vi "Configure Trigger (Logic).vi"(0 "VISA resource name":refnum<visa-resource-name>, 1 "Pattern Input":T1={"Channel 1 Logic Input (2: X)"=2, "Channel 2 Logic Input (2: X)"=2, "Channel 3 Logic Input (2: X)"=2, "Channel 4 Logic Input (2: X)"=2, "RF Channel Logic Input (2: X)"=2} {"RF Channel Logic Input (2: X)" items=["High", "Low", "X"]; "Channel 4 Logic Input (2: X)" items=["High", "Low", "X"]; "Channel 3 Logic Input (2: X)" items=["High", "Low", "X"]; "Channel 2 Logic Input (2: X)" items=["High", "Low", "X"]; "Channel 1 Logic Input (2: X)" items=["High", "Low", "X"]}, 2 "RF Logic Threshold (-22dBm)":dbl=-22.0 min=-40.0 max=10.0 step=1.0 format="%#_g dBm", 5 "Function (0: AND)":u16(ring) items=["AND", "OR", "NAND", "NOR"], 7 "Clock Source (1: Channel 1)":u16(ring)=1 items=["None", "Channel 1", "Channel 2", "Channel 3", "Channel 4", "Digital Channel 0", "Digital Channel 1", "Digital Channel 2", "Digital Channel 3", "Digital Channel 4", "Digital Channel 5", "Digital Channel 6", "Digital Channel 7", "Digital Channel 8", "Digital Channel 9", "Digital Channel 10", "Digital Channel 11", "Digital Channel 12", "Digital Channel 13", "Digital Channel 14", "Digital Channel 15", "RF"], 9 "Clock Polarity (0: Rising)":u16(ring) items=["Rising", "Falling"], 11 "error in (no error)":errorcluster, 12 "Trigger Condition (0: True)":u16(ring) items=["True", "False", "Less Than", "More Than", "Equal", "Not Equal"], 13 "Delta Time (4.0ns)":dbl=4e-09) -> (4 "VISA resource name out":refnum<visa-resource-name>, 15 "error out":errorcluster)   [LabVIEW 2013, in "Tektronix DPO MSO 2000 4000 Series.lvlib"]
doc: "Configures logic trigger settings for an oscilloscope."
uses:
  Tektronix DPO MSO 2000 4000 Series.lvlib
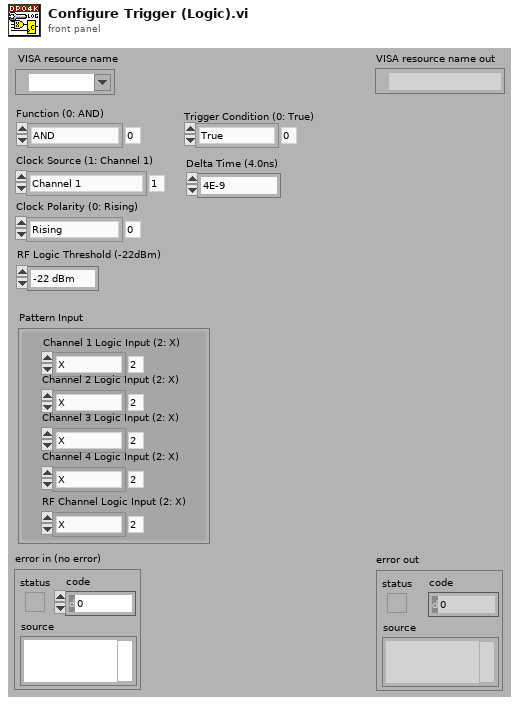
[diagram p1: front panel]
types:
  T1 = cluster{"Channel 1 Logic Input (2: X)":u16, "Channel 2 Logic Input (2: X)":u16, "Channel 3 Logic Input (2: X)":u16, "Channel 4 Logic Input (2: X)":u16, "RF Channel Logic Input (2: X)":u16}
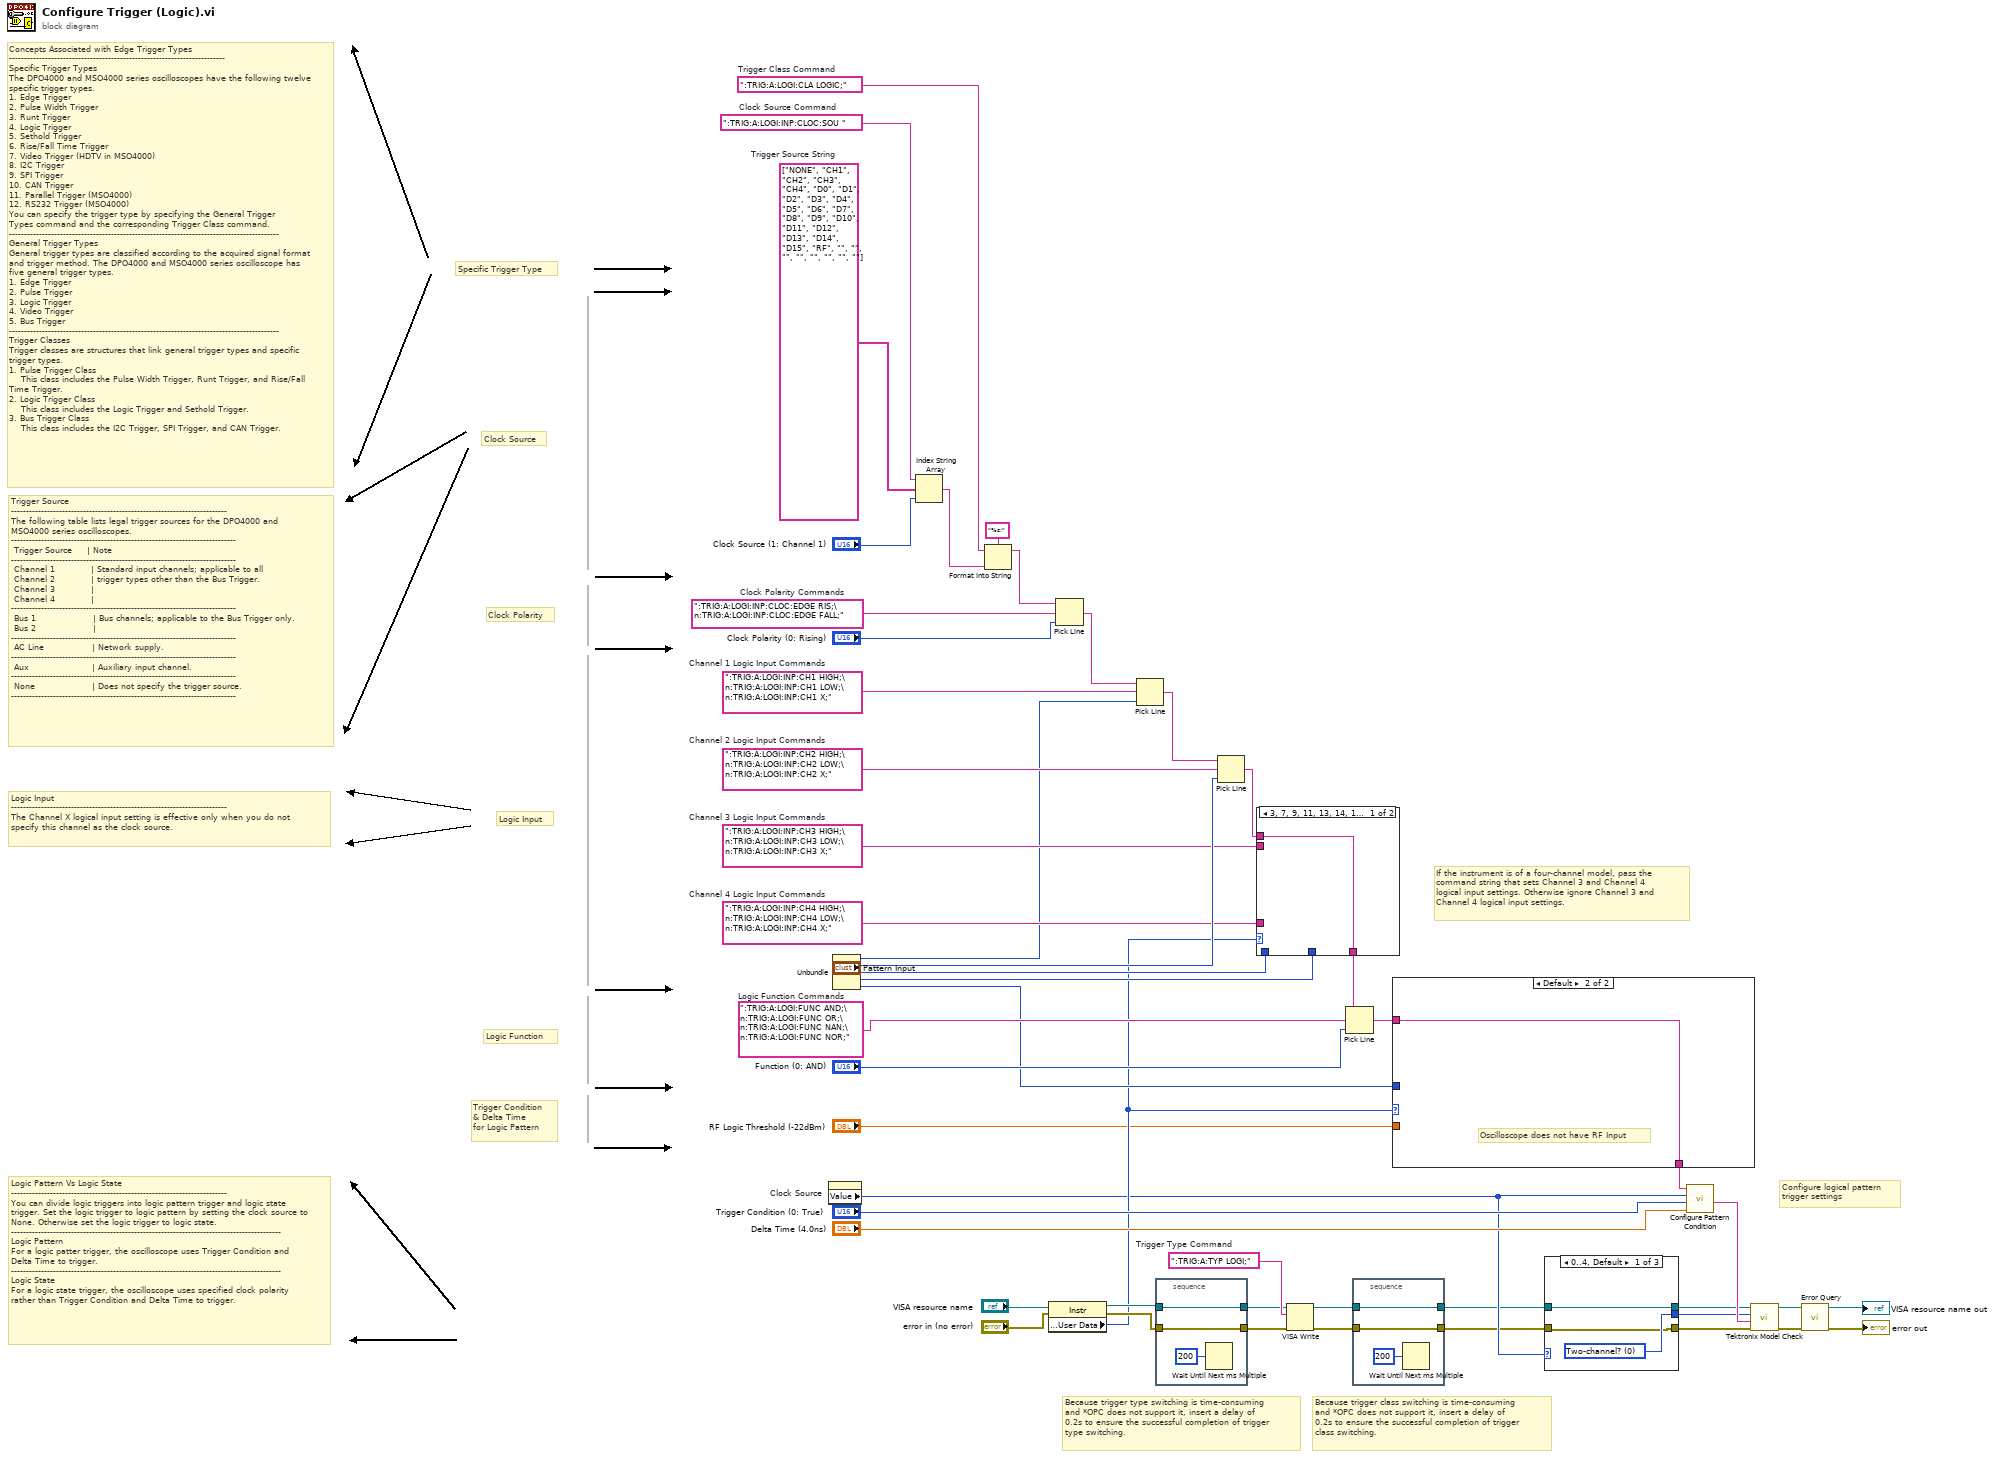
[diagram p0: block diagram]
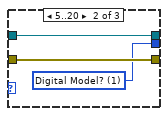
[diagram p2: hidden frame]
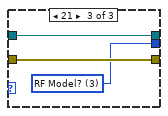
[diagram p3: hidden frame]
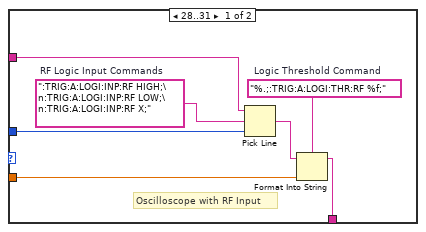
[diagram p4: hidden frame]
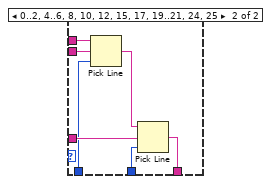
[diagram p5: hidden frame]
diagram:
  w25 = string[] ["NONE", "CH1", "CH2", "CH3", "CH4", "D0", "D1", "D2", "D3", "D4", "D5", "D6", "D7", "D8", "D9", "D10", "D11", "D12", "D13", "D14", "D15", "RF", "", "", "", "", "", "", "", ""]  # Trigger Source String
  w35 = ":TRIG:A:LOGI:INP:CH4 HIGH;\n:TRIG:A:LOGI:INP:CH4 LOW;\n:TRIG:A:LOGI:INP:CH4 X;"  # Channel 4 Logic Input Commands
  w36 = ":TRIG:A:LOGI:INP:CH3 HIGH;\n:TRIG:A:LOGI:INP:CH3 LOW;\n:TRIG:A:LOGI:INP:CH3 X;"  # Channel 3 Logic Input Commands
  w40 = ":TRIG:A:LOGI:INP:CH2 HIGH;\n:TRIG:A:LOGI:INP:CH2 LOW;\n:TRIG:A:LOGI:INP:CH2 X;"  # Channel 2 Logic Input Commands
  w41 = ":TRIG:A:LOGI:INP:CH1 HIGH;\n:TRIG:A:LOGI:INP:CH1 LOW;\n:TRIG:A:LOGI:INP:CH1 X;"  # Channel 1 Logic Input Commands
  w44 = ":TRIG:A:LOGI:FUNC AND;\n:TRIG:A:LOGI:FUNC OR;\n:TRIG:A:LOGI:FUNC NAN;\n:TRIG:A:LOGI:FUNC NOR;"  # Logic Function Commands
  w46 = ":TRIG:A:LOGI:INP:CLOC:EDGE RIS;\n:TRIG:A:LOGI:INP:CLOC:EDGE FALL;"  # Clock Polarity Commands
  w48 = ":TRIG:A:LOGI:INP:CLOC:SOU "  # Clock Source Command
  w24 = ":TRIG:A:LOGI:CLA LOGIC;"  # Trigger Class Command
  w51 = ":TRIG:A:TYP LOGI;"  # Trigger Type Command
  # "Trigger Source\n------------------------------------------------------------------------\nThe following table lists legal trigger sources for the DPO4000 and MSO4000 series oscilloscopes.\n---------------------------------------------------------------------------\n Trigger Source     | Note                                                           \n---------------------------------------------------------------------------\n Channel 1            | Standard input channels; applicable to all      \n Channel 2            | trigger types other than the Bus Trigger.         \n Channel 3            |     \n Channel 4            |\n---------------------------------------------------------------------------\n Bus 1                   | Bus channels; applicable to the Bus Trigger only.\n Bus 2                   | \n---------------------------------------------------------------------------\n AC Line                | Network supply.\n---------------------------------------------------------------------------\n Aux                     | Auxiliary input channel.\n---------------------------------------------------------------------------\n None                   | Does not specify the trigger source.\n---------------------------------------------------------------------------"
  # "Concepts Associated with Edge Trigger Types\n------------------------------------------------------------------------\nSpecific Trigger Types\nThe DPO4000 and MSO4000 series oscilloscopes have the following twelve specific trigger types.\n1. Edge Trigger\n2. Pulse Width Trigger\n3. Runt Trigger\n4. Logic Trigger\n5. Sethold Trigger\n6. Rise/Fall Time Trigger\n7. Video Trigger (HDTV in MSO4000)\n8. I2C Trigger\n9. SPI Trigger\n10. CAN Trigger\n11. Parallel Trigger (MSO4000)\n12. RS232 Trigger (MSO4000)\nYou can specify the trigger type by specifying the General Trigger \nTypes command and the corresponding Trigger Class command.\n------------------------------------------------------------------------------------------\nGeneral Trigger Types \nGeneral trigger types are classified according to the acquired signal format and trigger method. The DPO4000 and MSO4000 series oscilloscope has five general trigger types.\n1. Edge Trigger\n2. Pulse Trigger\n3. Logic Trigger\n4. Video Trigger\n5. Bus Trigger\n------------------------------------------------------------------------------------------\nTrigger Classes\nTrigger classes are structures that link general trigger types and specific trigger types.\n1. Pulse Trigger Class\n    This class includes the Pulse Width Trigger, Runt Trigger, and Rise/Fall Time Trigger.\n2. Logic Trigger Class\n    This class includes the Logic Trigger and Sethold Trigger.\n3. Bus Trigger Class\n    This class includes the I2C Trigger, SPI Trigger, and CAN Trigger."
  # "Because trigger type switching is time-consuming\nand *OPC does not support it, insert a delay of\n0.2s to ensure the successful completion of trigger\ntype switching."
  # "Because trigger class switching is time-consuming\nand *OPC does not support it, insert a delay of\n0.2s to ensure the successful completion of trigger\nclass switching."
  # "Configure logical pattern\ntrigger settings"
  # "If the instrument is of a four-channel model, pass the\ncommand string that sets Channel 3 and Channel 4\nlogical input settings. Otherwise ignore Channel 3 and\nChannel 4 logical input settings."
  # "Logic Pattern Vs Logic State\n------------------------------------------------------------------------\nYou can divide logic triggers into logic pattern trigger and logic state trigger. Set the logic trigger to logic pattern by setting the clock source to None. Otherwise set the logic trigger to logic state.\n------------------------------------------------------------------------------------------\nLogic Pattern\nFor a logic patter trigger, the oscilloscope uses Trigger Condition and Delta Time to trigger.\n------------------------------------------------------------------------------------------\nLogic State\nFor a logic state trigger, the oscilloscope uses specified clock polarity rather than Trigger Condition and Delta Time to trigger."
  # "Logic Input\n------------------------------------------------------------------------\nThe Channel X logical input setting is effective only when you do not specify this channel as the clock source."
  # "Trigger Condition\n& Delta Time \nfor Logic Pattern"
  # "Logic Function"
  # "Logic Input"
  # "Clock Polarity"
  # "Clock Source"
  # "Specific Trigger Type"
  n1 = property on="Clock Source" class="Ring (strict)"() -> ("Value"=w6:u16)  [unwired: 2 in, 2 out]
  n2 = Unbundle("Pattern Input") -> ("Channel 1 Logic Input (2: X)"=w16:u16, "Channel 2 Logic Input (2: X)"=w38:u16, "Channel 3 Logic Input (2: X)"=w34:u16, "Channel 4 Logic Input (2: X)"=w33:u16, "RF Channel Logic Input (2: X)"=w10:u16)
  n3 = Index String Array(1:"Clock Source (1: Channel 1)", 2:w25, 3:w48) -> (0:w23:string)
  n4 = Format Into String(format string="%s;", initial string=w24, w23) -> (resulting string=w45:string)  [unwired: 1 in, 1 out]
  n5 = property class="Instr"(reference="VISA resource name", error in="error in (no error)") -> (reference out=w21:refnum<visa-resource-name>, error out=w20:errorcluster, "General Settings:User Data"=w9:u32)
  n6 = Pick Line(string ("")=w45, multi-line string=w46, line index="Clock Polarity (0: Rising)") -> (output string=w22:string)
  n7 = Pick Line(string ("")=w22, multi-line string=w41, line index=w16) -> (output string=w39:string)
  n8 = stacked-sequence {
    tunnel: w21 -> [w53]
    tunnel: [w53] -> w50
    tunnel: w20 -> [w52]
    tunnel: [w52] -> w49
    frame #0 {
      n9 = Wait Until Next ms Multiple(millisecond multiple=u32 200) -> ()  [unwired: 1 out]
    }
  }
  n10 = Pick Line(string ("")=w39, multi-line string=w40, line index=w38) -> (output string=w37:string)
  n11 = case shown="3, 7, 9, 11, 13, 14, 16, 18, 22, 23, 26, 27, Default" w9 {
    tunnel: w37 -> [w55 w62]
    tunnel: w36 -> [_ w61]
    tunnel: w35 -> [_ w59]
    tunnel: w34 -> [_ w58]
    tunnel: w33 -> [_ w57]
    tunnel: [w55 w56] -> w17
    frame 3, 7, 9, 11, 13, 14, 16, 18, 22, 23, 26, 27, Default {
    }
    frame 0..2, 4..6, 8, 10, 12, 15, 17, 19..21, 24, 25 {
      n12 = Pick Line(string ("")=w62, multi-line string=w61, line index=w58) -> (output string=w60:string)
      n13 = Pick Line(string ("")=w60, multi-line string=w59, line index=w57) -> (output string=w56:string)
    }
  }
  n14 = VISA Write(VISA resource name=w50, write buffer=w51, error in (no error)=w49) -> (VISA resource name out=w32:refnum<visa-resource-name>, error out=w31:errorcluster)  [unwired: 1 out]
  n15 = Pick Line(string ("")=w17, multi-line string=w44, line index="Function (0: AND)") -> (output string=w11:string)
  n16 = stacked-sequence {
    tunnel: w32 -> [w64]
    tunnel: [w64] -> w5
    tunnel: w31 -> [w63]
    tunnel: [w63] -> w3
    frame #0 {
      n17 = Wait Until Next ms Multiple(millisecond multiple=u32 200) -> ()  [unwired: 1 out]
    }
  }
  n18 = case shown="Default" w9 {
    tunnel: w11 -> [w70 w73]
    tunnel: w10 -> [w71 _]
    tunnel: "RF Logic Threshold (-22dBm)" -> [w69 _]
    tunnel: [w66 w73] -> w7
    frame 28..31 {
      w67 = "%.;:TRIG:A:LOGI:THR:RF %f;"  # Logic Threshold Command
      w72 = ":TRIG:A:LOGI:INP:RF HIGH;\n:TRIG:A:LOGI:INP:RF LOW;\n:TRIG:A:LOGI:INP:RF X;"  # RF Logic Input Commands
      # "Oscilloscope with RF Input"
      n19 = Pick Line(string ("")=w70, multi-line string=w72, line index=w71) -> (output string=w68:string)
      n20 = Format Into String(format string=w67, initial string=w68, w69) -> (resulting string=w66:string)  [unwired: 1 in, 1 out]
    }
    frame Default {
      # "Oscilloscope does not have RF Input"
    }
  }
  n21 = case shown="0..4, Default" w6 {
    tunnel: w5 -> [w74 w79 w82]
    tunnel: [w74 w79 w82] -> w4
    tunnel: w3 -> [w75 w78 w81]
    tunnel: [w75 w78 w81] -> w2
    tunnel: [w76 w77 w80] -> w1
    frame 0..4, Default {
      w76 = u16 0 items=["Two-channel?", "Digital Model?", "Four-channel?", "RF Model?"] ("Oscilloscope Model Tests (3: RF Model?)")
    }
    frame 5..20 {
      w77 = u16 1 items=["Two-channel?", "Digital Model?", "Four-channel?", "RF Model?"] ("Oscilloscope Model Tests (3: RF Model?)")
    }
    frame 21 {
      w80 = u16 3 items=["Two-channel?", "Digital Model?", "Four-channel?", "RF Model?"] ("Oscilloscope Model Tests (3: RF Model?)")
    }
  }
  n22 = call "Configure Pattern Condition.vi"("Delta Time (2.5E-9)"="Delta Time (4.0ns)", "Trigger Condition (0: True)"="Trigger Condition (0: True)", "Clock Source (0: Channel 1)"=w6, "Input Command String"=w7) -> ("Output Command String"=w14:string)  [unwired: 7 in]
  n23 = call "Tektronix Model Check.vi"("error in (no error)"=w2, "Command String"=w14, "Oscilloscope Model Tests (3: RF Model?)"=w1, "VISA resource name"=w4) -> ("error out"=w12:errorcluster, "VISA resource name out"=w13:refnum<visa-resource-name>)  [unwired: 6 in]
  n24 = call "Error Query.vi"("error in (no error)"=w12, "VISA resource name"=w13) -> ("error out"=→"error out":errorcluster, "VISA resource name out"=→"VISA resource name out":refnum<visa-resource-name>)  [unwired: 6 in, 2 out]
